vi "Initialize Plot Porperty Page.vi"(6 "Plot Area Ref":refnum<vi>, 8 "error in (no error)":errorcluster, 9 "2D Featherr Array In":T3, 11 "Plot Property Array In":T1) -> (0 "error out":errorcluster, 1 "2D Feather Array Out":T3, 3 "Plot Property Array Out":T1)   [LabVIEW 2017, in "2D Feather.lvclass"]
uses:
  <vilib>/Math Plots/2D Math Plots/2D Feather/2D Feather/2D Feather.lvclass
  <vilib>/Math Plots/2D Math Plots/2D Feather/2D Feather/Typedef/2D Feather Property Array.ctl
  <vilib>/Math Plots/2D Math Plots/2D Feather/2D Feather/Typedef/2D Feather Property.ctl
  <vilib>/Math Plots/2D Math Plots/2D Plot/2D Plot/Typedef/Plot Property Array.ctl
  <vilib>/Math Plots/2D Math Plots/2D Plot/2D Plot/Typedef/Plot Property.ctl
  <vilib>/Math Plots/2D Math Plots/2D Plot/2D Plot/2D Plot.lvclass
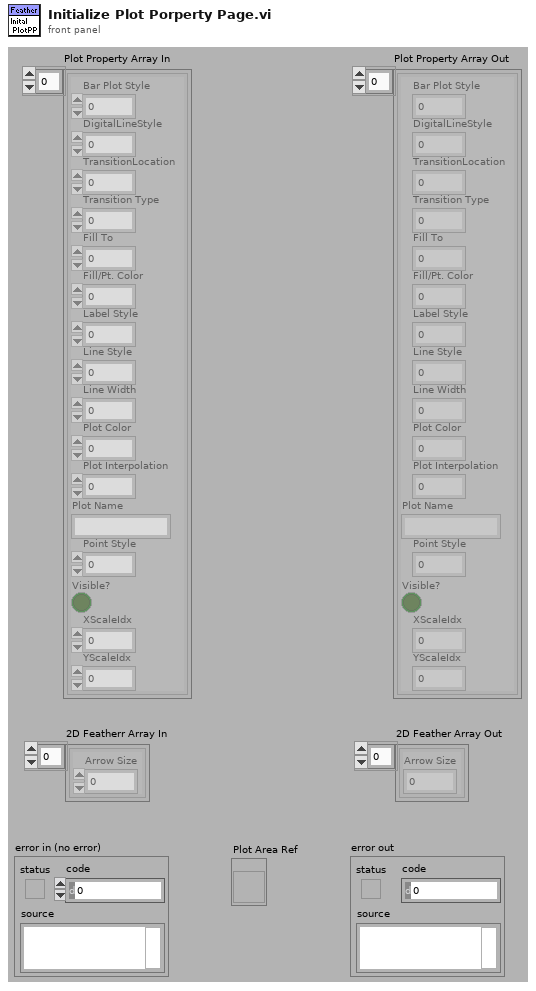
[diagram p1: front panel]
types:
  T1 = typedef "2D Plot.lvclass/Plot Property Array.ctl" = T2[]
  T2 = typedef "2D Plot.lvclass/Plot Property.ctl" = cluster{"Bar Plot Style":u8, "DigitalLineStyle":u8, "TransitionLocation":u8, "Transition Type":u8, "Fill To":i16, "Fill/Pt. Color":u32, "Label Style":u8, "Line Style":u8, "Line Width":u8, "Plot Color":u32, "Plot Interpolation":u8, "Plot Name":string, "Point Style":u8, "Visible?":bool, "XScaleIdx":u32, "YScaleIdx":u32}
  T3 = typedef "2D Feather.lvclass/2D Feather Property Array.ctl" = T4[]
  T4 = typedef "2D Feather.lvclass/2D Feather Property.ctl" = cluster{"Arrow Size":dbl}
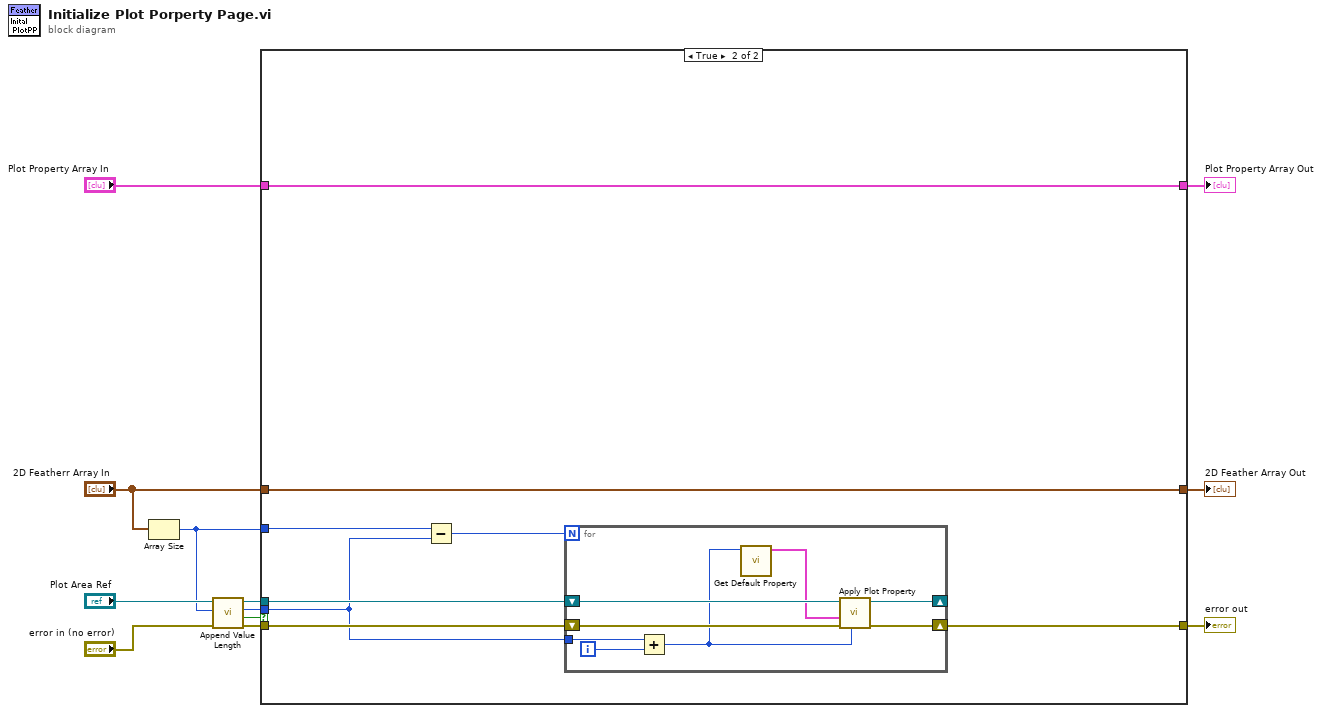
[diagram p0: block diagram]
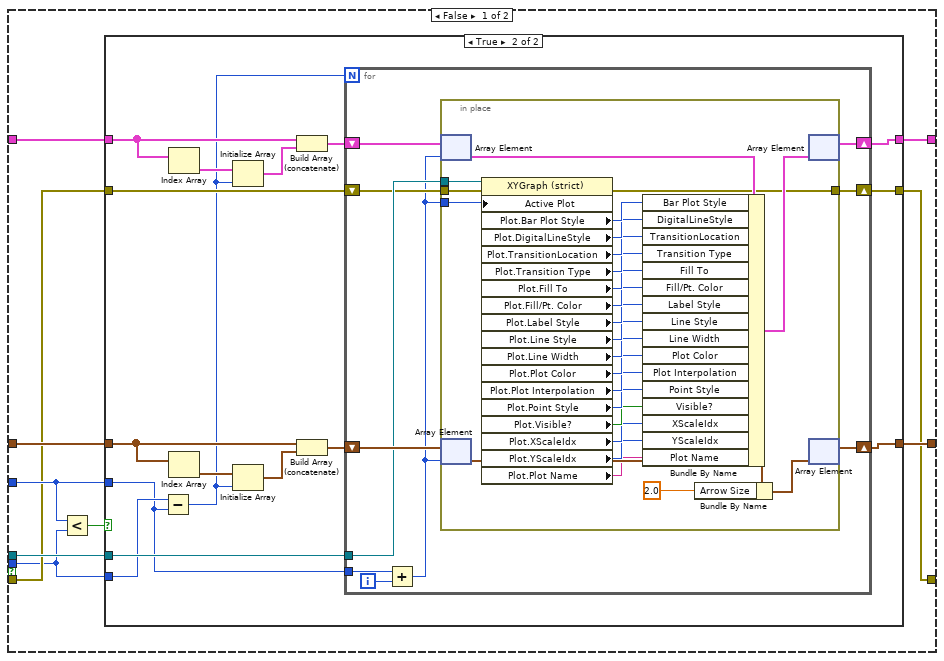
[diagram p2: hidden frame]
diagram:
  n1 = Array Size(array="2D Featherr Array In") -> (size(s)=w5:i32)
  n2 = call <vilib>:"Append Value Length.vi"("error in (no error)"="error in (no error)", "Expect Value Length"=w5, "Plot Area Ref In"="Plot Area Ref") -> ("error out"=w2:errorcluster, "Append Value?"=w4:bool, "Actual Value Length"=w1:i32, "Plot Area Ref Out"=w3:refnum<vi>)  [unwired: 1 in, 4 out]
  n3 = case shown="True" w4 {
    tunnel: "Plot Property Array In" -> [w21 w84]
    tunnel: [w22 w84] -> w11
    tunnel: "2D Featherr Array In" -> [w19 w83]
    tunnel: [w20 w83] -> w12
    tunnel: w3 -> [w17 w79]
    tunnel: w5 -> [w16 w82]
    tunnel: w2 -> [w15 w78]
    tunnel: [w14 w81] -> w8
    tunnel: w1 -> [w13 w77]
    frame False {
      n4 = Less?(x=w16, y=w13) -> (x < y?=w18:bool)
      n5 = case shown="True" w18 {
        tunnel: [w25 w34] -> w22
        tunnel: w21 -> [w25 w37]
        tunnel: [w24 w33] -> w20
        tunnel: w19 -> [w24 w29]
        tunnel: w17 -> [_ w41]
        tunnel: w16 -> [_ w35]
        tunnel: w13 -> [_ w40]
        tunnel: w15 -> [w23 w28]
        tunnel: [w23 w27] -> w14
        frame False {
        }
        frame True {
          n6 = Subtract(x=w40, y=w35) -> (x-y=w26:i32)
          n7 = Index Array(array=w37) -> (element=w39:T2)  [unwired: 1 in]
          n8 = Index Array(array=w29) -> (element=w31:T4)  [unwired: 1 in]
          n9 = Initialize Array(w39, w26) -> (w38:T2[])
          n10 = Initialize Array(w31, w26) -> (w32:T4[])
          n11 = Build Array (concatenate)(w37, w38) -> (w36:T1)
          n12 = Build Array (concatenate)(w29, w32) -> (w30:T3)
          n13 = for {
            N: w26 -> [_]
            tunnel: w41 -> [w45]
            tunnel: w35 -> [w51]
            shift-right: [w48] -> w34
            shift-left: w36 -> [w49]
            shift-right: [w47] -> w33
            shift-left: w30 -> [w50]
            shift-right: [w43] -> w27
            shift-left: w28 -> [w44]
            i -> [w46]
            n14 = Add(x=w51, y=w46) -> (x+y=w42:i32)
            n15 = in-place {
              in-place-border: w45 -> [w71]
              in-place-border: w42 -> [w70]
              in-place-border: w44 -> [w54]
              in-place-border: [w53] -> w43
              n16 = in-place-array #1(w49, w42) -> (w76:T2)
              n17 = in-place-array #2(w50, w42) -> (w74:T4)
              n18 = property class="XYGraph (strict)"(reference=w71, error in=w54, "Active Plot"=w70) -> (error out=w53:errorcluster, "Plot.Bar Plot Style"=w69:u8, "Plot.DigitalLineStyle"=w68:u8, "Plot.TransitionLocation"=w67:u8, "Plot.Transition Type"=w66:u8, "Plot.Fill To"=w65:i16, "Plot.Fill/Pt. Color"=w64:u32, "Plot.Label Style"=w63:u8, "Plot.Line Style"=w62:u8, "Plot.Line Width"=w61:u8, "Plot.Plot Color"=w60:u32, "Plot.Plot Interpolation"=w59:u8, "Plot.Point Style"=w58:u8, "Plot.Visible?"=w57:bool, "Plot.XScaleIdx"=w56:u32, "Plot.YScaleIdx"=w55:u32, "Plot.Plot Name"=w52:string)  [unwired: 1 out]
              n19 = Bundle By Name(cluster=w76, "Bar Plot Style"=w69, "DigitalLineStyle"=w68, "TransitionLocation"=w67, "Transition Type"=w66, "Fill To"=w65, "Fill/Pt. Color"=w64, "Label Style"=w63, "Line Style"=w62, "Line Width"=w61, "Plot Color"=w60, "Plot Interpolation"=w59, "Point Style"=w58, "Visible?"=w57, "XScaleIdx"=w56, "YScaleIdx"=w55, "Plot Name"=w52) -> (w75:T2)
              n20 = Bundle By Name(cluster=w74, "Arrow Size"=2.0) -> (w73:T4)
              n21 = in-place-array #1(w75) -> (w48:T1)  [unwired: 1 out]
              n22 = in-place-array #2(w73) -> (w47:T3)  [unwired: 1 out]
            }
          }
        }
      }
    }
    frame True {
      n23 = Subtract(x=w82, y=w77) -> (x-y=w80:i32)
      n24 = for {
        N: w80 -> [_]
        tunnel: w77 -> [w90]
        shift-right: [w92] -> w81
        shift-left: w78 -> [w87]
        shift-right: [w89] -> _
        shift-left: w79 -> [w88]
        i -> [w91]
        n25 = Add(x=w90, y=w91) -> (x+y=w86:i32)
        n26 = call <vilib>:"Get Default Property.vi"("Index"=w86) -> ("Temporary Property"=w85:T2)  [unwired: 3 in, 7 out]
        n27 = call <vilib>:"Apply Plot Property.vi"("Plot ID"=w86, "error in (no error)"=w87, "Plot Property"=w85, "Polar Area Ref In"=w88) -> ("error out"=w92:errorcluster, "Polar Area Ref Out"=w89:refnum<vi>)  [unwired: 1 in, 5 out]
      }
    }
  }
  "2D Feather Array Out" <- w12
  "Plot Property Array Out" <- w11
  "error out" <- w8
